vi "WS105x Stress Beams.vi"(8 "error in (no error)":errorcluster, 11 "Cycling Bit":string[](array[string])=["0702013B3B3B", "070201000000"]) -> (0 "error out":errorcluster, 2 "Cmd":string, 3 "Beams":string)   [LabVIEW 2012]
uses:
  <vilib>/Utility/error.llb/whitespace.ctl
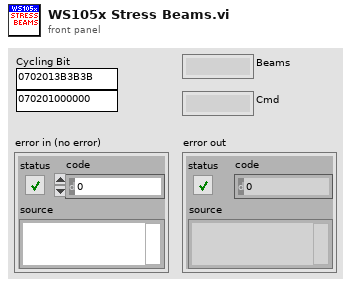
[diagram p1: front panel]
types:
  T1 = typedef "whitespace.ctl" = u16
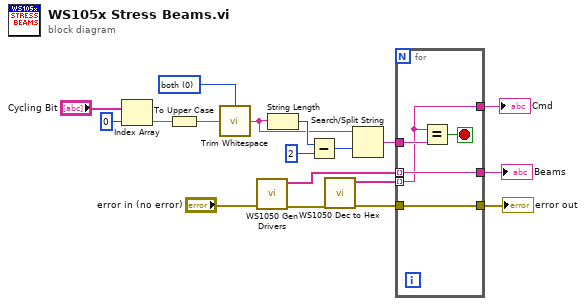
[diagram p0: block diagram]
diagram:
  w16 = T1 0 items=["both", "start of string", "end of string"] ("location (both)")
  n1 = Index Array(array="Cycling Bit", index=0) -> (element=w2:string)
  n2 = To Upper Case(1:w2) -> (0:w1:string)
  n3 = call <vilib>:"Trim Whitespace.vi"("string"=w1, "location (both)"=w16) -> ("trimmed string"=w12:string)
  n4 = call "WS1050 Gen Drivers.vi"("error in (no error)"="error in (no error)") -> ("error out"=w7:errorcluster, "WS1050 Drivers"=w5:string[])  [unwired: 9 in]
  n5 = String Length(string=w12) -> (length=w15:i32)
  n6 = Subtract(x=w15, y=2) -> (x-y=w13:i32)
  n7 = call "WS1050 Dec to Hex.vi"("error in (no error)"=w7) -> ("error out"=w6:errorcluster, "Hex"=w3:string[])  [unwired: 9 in]
  n8 = Search/Split String(string=w12, offset (0)=w13) -> (match + rest of string=w11:string)  [unwired: 1 in, 2 out]
  n9 = for {
    tunnel: w11 -> [w23]
    tunnel: [w19] -> w10
    tunnel: w6 -> [w21]
    tunnel: [w21] -> w9
    tunnel: w5 -> [w20] mode=indexing
    tunnel: [w20] -> w4
    tunnel: w3 -> [w19] mode=indexing
    stop <- w22 stop-if-true
    n10 = Equal?(x=w19, y=w23) -> (x = y?=w22:bool)
  }
  "Beams" <- w4
  "Cmd" <- w10
  "error out" <- w9
